vi "ProductRequest.vi"(8 "error in (no error)":errorcluster, 10 "Product Info":cluster{"Name":string, "Price":dbl, "Stock":i32}, 11 "Messages Actor in":refnum<class "Messages Actor.lvclass">) -> (0 "error out":errorcluster, 3 "Messages Actor out":refnum<class "Messages Actor.lvclass">)   [LabVIEW 2020, in "Messages Actor.lvlib" / "Messages Actor.lvclass"]
uses:
  Messages Actor.lvclass
  C:/Program Files (x86)/National Instruments/LabVIEW 2020/vi.lib/ActorFramework/Actor/Actor.lvclass
  <vilib>/ActorFramework/Actor/Actor.lvclass/Actor.ctl
  <vilib>/ActorFramework/Message Enqueuer/Message Enqueuer.lvclass/Message Enqueuer.ctl
  Messages Actor.lvclass/Messages Actor.ctl
  Messages Actor Messages/Product Selected Msg/Product Selected Msg.lvclass/Product Selected Msg.ctl
  Messages Actor Messages/UpdateChange Msg/UpdateChange Msg.lvclass/UpdateChange Msg.ctl
  <vilib>/ActorFramework/Message Enqueuer/Init from Existing Queue.vi
  <vilib>/ActorFramework/Message Enqueuer/Enqueue.vi
  Messages Actor Messages/Product Selected Msg/Product Selected Msg.lvclass
  C:/Program Files (x86)/National Instruments/LabVIEW 2020/vi.lib/ActorFramework/Message/Message.lvclass
  Messages Actor Messages/UpdateChange Msg/UpdateChange Msg.lvclass
  Messages Actor Messages/ResetCredit Msg/ResetCredit Msg.lvclass
  UI Actor Messages/UpdateProducts Msg/UpdateProducts Msg.lvclass
  <vilib>/ActorFramework/Message Priority Queue/Priority Enqueue.vi
  <vilib>/ActorFramework/Message Enqueuer/Message Enqueuer.lvclass
  <vilib>/ActorFramework/Actor/Actor.lvclass
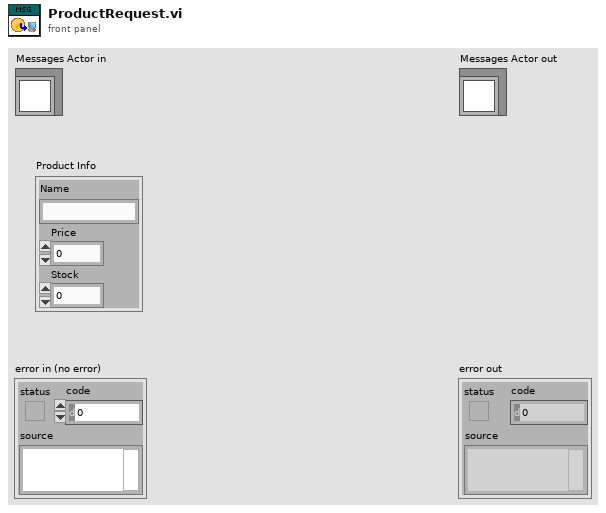
[diagram p1: front panel]
types:
  T1 = typedef "Language Enum.ctl" = enum16{"English", "Español", "Français"}
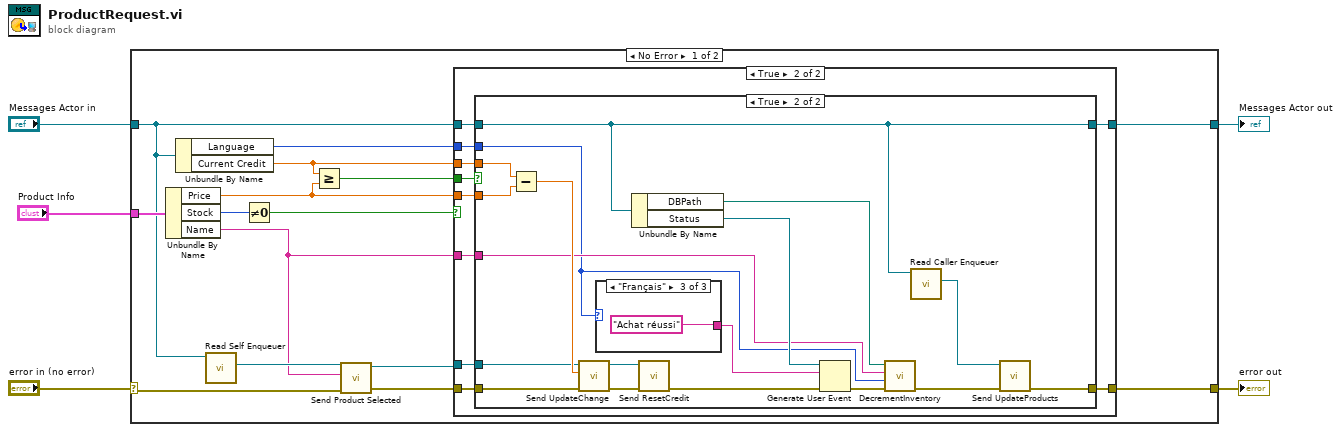
[diagram p0: block diagram]
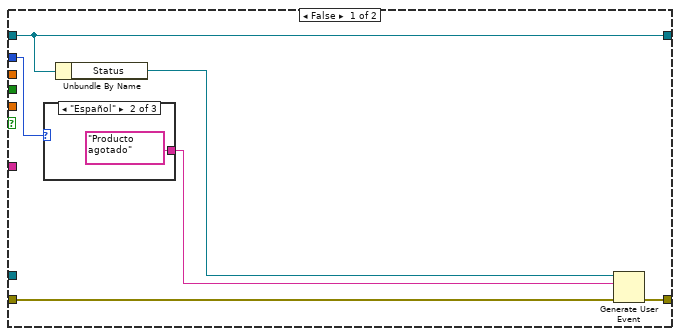
[diagram p2: hidden frame]
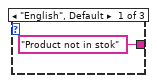
[diagram p3: hidden frame]
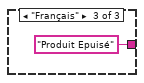
[diagram p4: hidden frame]
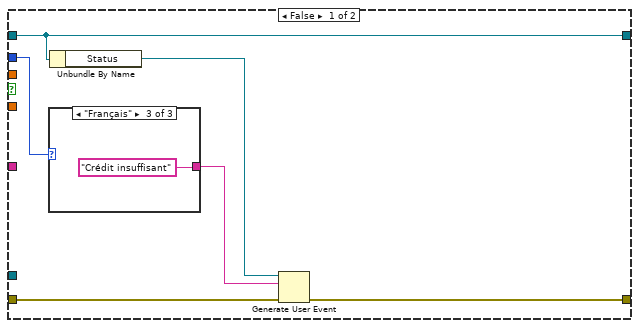
[diagram p5: hidden frame]
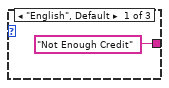
[diagram p6: hidden frame]
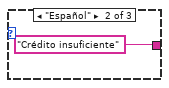
[diagram p7: hidden frame]
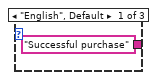
[diagram p8: hidden frame]
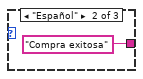
[diagram p9: hidden frame]
diagram:
  n1 = case shown="No Error" "error in (no error)" {
    selector: "error in (no error)" -> [w8 w71]
    tunnel: [w19 w71] -> w4
    tunnel: [w18 w70] -> w2
    tunnel: "Messages Actor in" -> [w13 w70]
    tunnel: "Product Info" -> [w20 _]
    frame No Error {
      n2 = Unbundle By Name(w20) -> ("Price"=w11:dbl, "Stock"=w16:i32, "Name"=w6:string)
      n3 = Unbundle By Name(w13) -> ("Language"=w14:T1, "Current Credit"=w12:dbl)
      n4 = call <vilib>:"Read Self Enqueuer.vi"("Actor"=w13) -> ("Self Enqueuer"=w7:refnum<class "Message Enqueuer.lvclass">)  [unwired: 10 in]
      n5 = Not Equal To 0?(x=w16) -> (x != 0?=w15:bool)
      n6 = Greater Or Equal?(x=w12, y=w11) -> (x >= y?=w17:bool)
      n7 = call "Send Product Selected.vi"("error in (no error)"=w8, "Product"=w6, "Message Enqueuer"=w7) -> ("error out"=w9:errorcluster, "Message Enqueuer out"=w10:refnum<class "Message Enqueuer.lvclass">)  [unwired: 7 in]
      n8 = case shown="True" w15 {
        tunnel: w9 -> [w26 w39]
        tunnel: [w24 w38] -> w19
        tunnel: w13 -> [w25 w37]
        tunnel: [w25 w36] -> w18
        tunnel: w17 -> [_ w35]
        tunnel: w14 -> [w22 w31]
        tunnel: w12 -> [_ w34]
        tunnel: w11 -> [_ w33]
        tunnel: w10 -> [_ w32]
        tunnel: w6 -> [_ w30]
        frame False {
          n9 = case shown="\"Español\"" w22 {
            tunnel: ["Product not in stok" ("event data") "Producto agotado" ("event data") "Produit Epuisé" ("event data")] -> w21
            frame "English", Default {
            }
            frame "Español" {
            }
            frame "Français" {
            }
          }
          n10 = Unbundle By Name(w25) -> ("Status"=w23:refnum<user-event>)
          n11 = Generate User Event(user event=w23, event data cluster=w21, error in=w26) -> (error out=w24:errorcluster)  [unwired: 1 in, 1 out]
        }
        frame True {
          n12 = case shown="True" w35 {
            tunnel: w39 -> [w45 w62]
            tunnel: [w44 w56] -> w38
            tunnel: w37 -> [w43 w57]
            tunnel: [w43 w57] -> w36
            tunnel: w34 -> [_ w65]
            tunnel: w33 -> [_ w64]
            tunnel: w32 -> [_ w60]
            tunnel: w31 -> [w41 w50]
            tunnel: w30 -> [_ w51]
            frame False {
              n13 = case shown="\"Français\"" w41 {
                tunnel: ["Not Enough Credit" ("event data") "Crédito insuficiente" ("event data") "Crédit insuffisant" ("event data")] -> w40
                frame "English", Default {
                }
                frame "Español" {
                }
                frame "Français" {
                }
              }
              n14 = Unbundle By Name(w43) -> ("Status"=w42:refnum<user-event>)
              n15 = Generate User Event(user event=w42, event data cluster=w40, error in=w45) -> (error out=w44:errorcluster)  [unwired: 1 in, 1 out]
            }
            frame True {
              n16 = Subtract(x=w65, y=w64) -> (x-y=w61:dbl)
              n17 = call "Send UpdateChange.vi"("error in (no error)"=w62, "Change"=w61, "Message Enqueuer"=w60) -> ("error out"=w63:errorcluster, "Message Enqueuer out"=w59:refnum<class "Message Enqueuer.lvclass">)  [unwired: 7 in]
              n18 = case shown="\"Français\"" w50 {
                tunnel: ["Successful purchase" "Compra exitosa" "Achat réussi"] -> w58
                frame "English", Default {
                }
                frame "Español" {
                }
                frame "Français" {
                }
              }
              n19 = Unbundle By Name(w57) -> ("DBPath"=w49:path, "Status"=w52:refnum<user-event>)
              n20 = call "Send ResetCredit.vi"("error in (no error)"=w63, "Message Enqueuer"=w59) -> ("error out"=w66:errorcluster)  [unwired: 8 in, 1 out]
              n21 = Generate User Event(user event=w52, event data cluster=w58, error in=w66) -> (error out=w54:errorcluster)  [unwired: 1 in, 1 out]
              n22 = call "DecrementInventory.vi"("error in"=w54, "Language"=w50, "Name"=w51, "DB Path"=w49) -> ("error out"=w53:errorcluster)  [unwired: 7 in]
              n23 = call <vilib>:"Read Caller Enqueuer.vi"("Actor"=w57) -> ("Caller Enqueuer"=w55:refnum<class "Message Enqueuer.lvclass">)  [unwired: 10 in]
              n24 = call "Send UpdateProducts.vi"("error in (no error)"=w53, "Message Enqueuer"=w55) -> ("error out"=w56:errorcluster)  [unwired: 8 in, 1 out]
            }
          }
        }
      }
    }
    frame Error {
    }
  }
  "error out" <- w4
  "Messages Actor out" <- w2
